vi "Pop Up Message.vi"(4 "Text Settings":T1={"Minimum Size (15)"=15, "Maximum Size (45)"=45, "Bold?"=FALSE}, 6 "Message":string, 7 "Title":string, 8 "error in (no error)":errorcluster, 9 "Button Labels":string[](array[string]), 10 "Configuration":T2(tab), 11 "Test Class in":refnum<class "Test Class.lvclass">) -> (0 "error out":errorcluster, 2 "Button Pressed":string, 3 "Test Class out":refnum<class "Test Class.lvclass">)   [LabVIEW 2015, in "Test Class.lvclass"]
uses:
  Test Class.lvclass
  PopUp Text Settings.ctl
panel:
  in  "Message":string
  in  "1 Button - Button 1":bool=TRUE
  in  "2 Button - Button 1":bool=TRUE
  in  "2 Button - Button 2":bool=TRUE
  in  "3 Button - Button 3":bool=TRUE
  in  "3 Button - Button 2":bool=TRUE
  in  "3 Button - Button 1":bool=TRUE
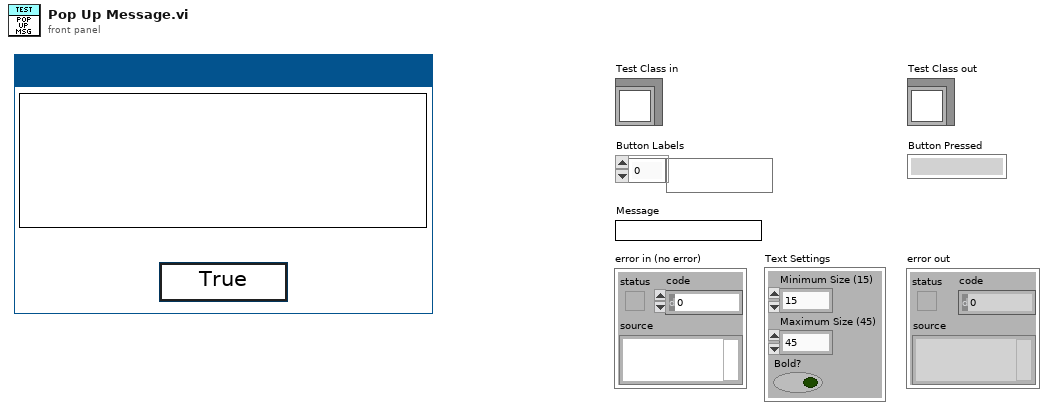
[diagram p1: front panel]
types:
  T1 = typedef "Test Class.lvclass/PopUp Text Settings.ctl" = cluster{"Minimum Size (15)":i16, "Maximum Size (45)":i16, "Bold?":bool}
  T2 = enum32{"One Button", "Two Button", "Three Button"}
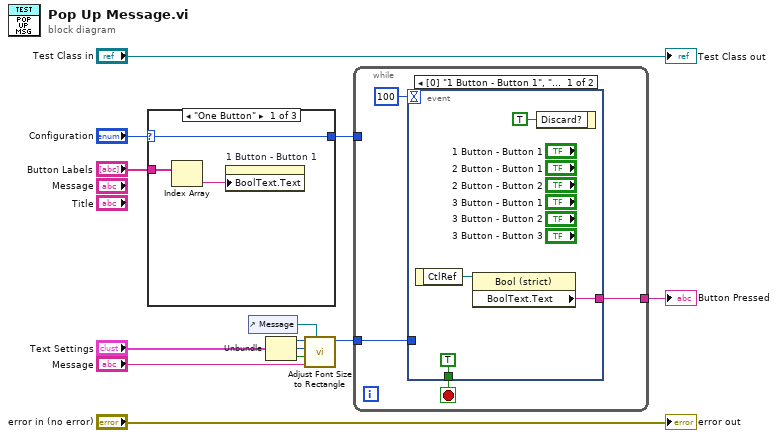
[diagram p0: block diagram]
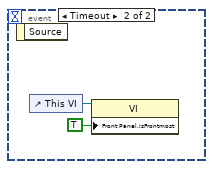
[diagram p2: hidden frame]
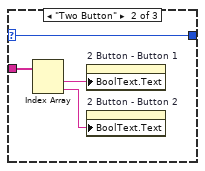
[diagram p3: hidden frame]
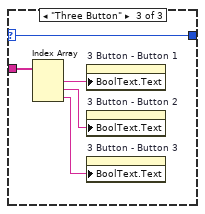
[diagram p4: hidden frame]
diagram:
  n1 = case shown="\"One Button\"" "Configuration" {
    selector: "Configuration" -> [w14 w17 w21]
    tunnel: "Button Labels" -> [w16 w20 w25]
    tunnel: [w14 w17 w21] -> w2
    frame "One Button" {
      n2 = Index Array(array=w16) -> (element=w15:string)  [unwired: 1 in]
      n3 = property on="1 Button - Button 1" class="Bool (strict)"("BoolText.Text"=w15) -> ()  [unwired: 2 in, 2 out]
    }
    frame "Two Button" {
      n4 = Index Array(array=w20) -> (element #1=w19:string, element #2=w18:string)  [unwired: 2 in]
      n5 = property on="2 Button - Button 1" class="Bool (strict)"("BoolText.Text"=w19) -> ()  [unwired: 2 in, 2 out]
      n6 = property on="2 Button - Button 2" class="Bool (strict)"("BoolText.Text"=w18) -> ()  [unwired: 2 in, 2 out]
    }
    frame "Three Button" {
      n7 = Index Array(array=w25) -> (element #1=w24:string, element #2=w23:string, element #3=w22:string)  [unwired: 3 in]
      n8 = property on="3 Button - Button 1" class="Bool (strict)"("BoolText.Text"=w24) -> ()  [unwired: 2 in, 2 out]
      n9 = property on="3 Button - Button 2" class="Bool (strict)"("BoolText.Text"=w23) -> ()  [unwired: 2 in, 2 out]
      n10 = property on="3 Button - Button 3" class="Bool (strict)"("BoolText.Text"=w22) -> ()  [unwired: 2 in, 2 out]
    }
  }
  n11 = control-ref of="Message"() -> (w11:refnum<vi>)
  n12 = Unbundle("Text Settings") -> ("Minimum Size (15)"=w8:i16, "Maximum Size (45)"=w7:i16, "Bold?"=w6:bool)
  n13 = call "Adjust Font Size to Rectangle.vi"("String Control Reference"=w11, "Message"="Message", "Bold?"=w6, "Maximum Size (45)"=w7, "Minimum Size (15)"=w8) -> ("Font Size"=w3:u32)  [unwired: 6 in]
  n14 = while {
    tunnel: w3 -> [w29]
    tunnel: w2 -> [_]
    tunnel: [w26] -> w1
    stop <- w27 stop-if-true
    n15 = event shown="[0] \"1 Button - Button 1\", \"2 Button - Button 1\", \"2 Button - Button 2\", \"3 Button - Button 1\", \"3 Button - Button 2\", \"3 Button - Button 3\": Mouse Down?" {
      selector: _ -> [_ _]
      dyn-events: _ -> [_ _]
      timeout: 100 -> [_ _]
      tunnel: w29 -> [_ _]
      tunnel: [TRUE _] -> w27
      tunnel: [w30 _] -> w26
      event "1 Button - Button 1", "2 Button - Button 1", "2 Button - Button 2", "3 Button - Button 1", "3 Button - Button 2", "3 Button - Button 3": Mouse Down? {
        n16 = event-data() -> ("CtlRef"=w31:refnum<vi>)  [unwired: 1 in]
        n17 = property on="Property Node" class="Bool (strict)"(reference=w31) -> ("BoolText.Text"=w30:string)  [unwired: 1 in, 2 out]
        n18 = event-data("Discard?"=TRUE) -> ()  [unwired: 1 in, 1 out]
      }
      event Timeout {
        n19 = event-data() -> ()  [unwired: 1 in, 1 out]
        n20 = control-ref of="This VI"() -> (w35:refnum<vi>)
        n21 = property class="VI"(reference=w35, "Front Panel.IsFrontmost"=TRUE ("Front Panel Window:Is Frontmost")) -> ()  [unwired: 1 in, 2 out]
      }
    }
  }
  "Button Pressed" <- w1
  "error out" <- "error in (no error)"
  "Test Class out" <- "Test Class in"
